vi "variantCtrlIoAddress.vi"(4 "isRequired (T)":bool=TRUE, 6 "menu in (get)":enum16{"get", "set"}(ring), 8 "error in":errorcluster, 9 "ADDR":T1 format="%04d", 11 "variant in":variant) -> (0 "error out":errorcluster, 1 "ADDR":T1 format="%04d", 2 "isFound?":bool, 3 "variant out":variant)   [LabVIEW 2024]
uses:
  controls/type.address.ctl
  controls/typeEngErrorCodes.ctl
panel:
  out "spreadsheet string":string
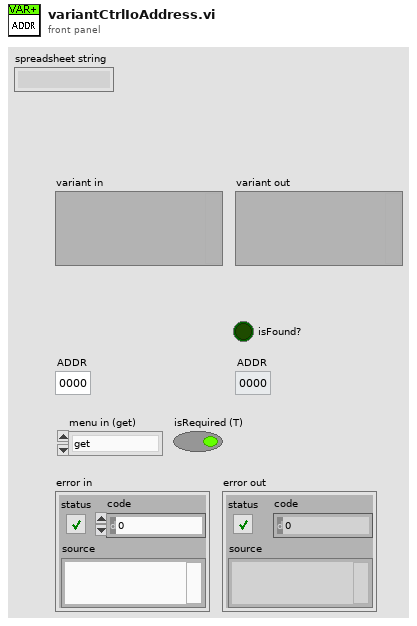
[diagram p1: front panel]
types:
  T1 = typedef "type.address.ctl" = u16
  T2 = typedef "typeEngErrorCodes.ctl" = u16
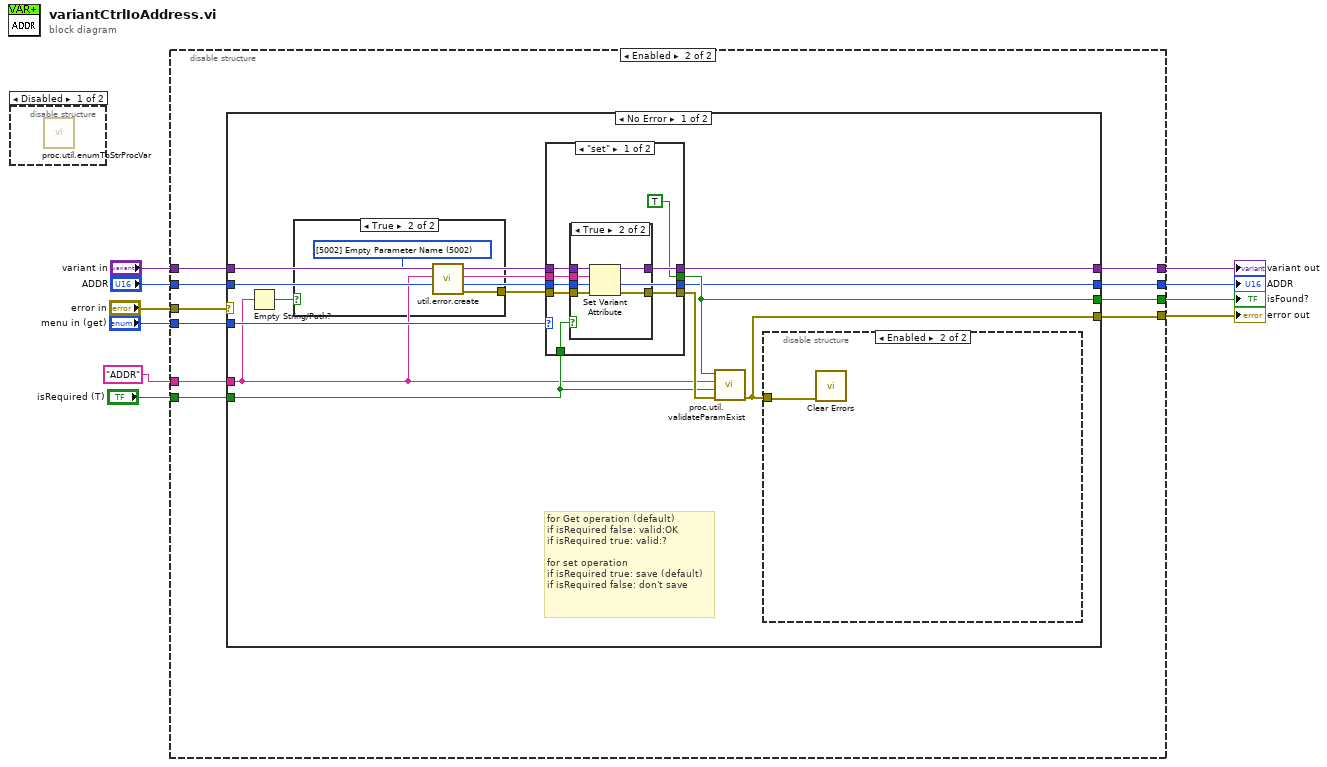
[diagram p0: block diagram]
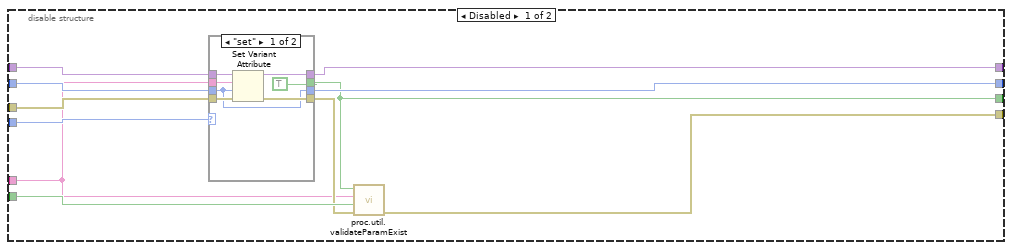
[diagram p2: hidden frame]
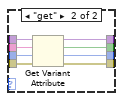
[diagram p3: hidden frame]
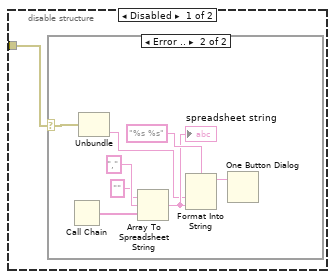
[diagram p5: hidden frame]
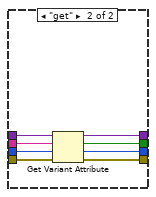
[diagram p8: hidden frame]
diagram:
  n1 = disable-structure shown="Disabled" {
    frame Disabled {
      n2 = call "proc.util.enumToStrProcVar.vi"() -> ()  [unwired: 11 in, 1 out]
    }
    frame Enabled {
    }
  }
  n3 = disable-structure shown="Enabled" {
    disable-tunnel: "error in" -> [w21 w43]
    disable-tunnel: "ADDR" -> [w20 w42]
    disable-tunnel: "variant in" -> [w19 w41]
    disable-tunnel: [w18 w40] -> w7
    disable-tunnel: "menu in (get)" -> [w17 w44]
    disable-tunnel: [w16 w38] -> w5
    disable-tunnel: "isRequired (T)" -> [w15 w45]
    disable-tunnel: [w14 w39] -> w3
    disable-tunnel: [w12 w37] -> w2
    disable-tunnel: "ADDR" ("name in") -> [w11 w46]
    frame Disabled {
      n4 = case shown="\"set\"" w17 {
        tunnel: w21 -> [w28 w36]
        tunnel: w20 -> [w23 w35]
        tunnel: w19 -> [w27 w34]
        tunnel: [w26 w33] -> w13
        tunnel: [TRUE w32] -> w14
        tunnel: [w25 w31] -> w18
        tunnel: w11 -> [w24 w30]
        tunnel: [w23 w29] -> w16
        frame "set" {
          n5 = Set Variant Attribute(Variant=w27, name=w24, value=w23, error in=w28) -> (Variant out=w25:variant, error out=w26:errorcluster)  [unwired: 1 out]
        }
        frame "get" {
          n6 = Get Variant Attribute(Variant=w34, name=w30, default value (empty Variant)=w35, error in=w36) -> (duplicate Variant=w31:variant, found=w32:bool, value=w29:T1, error out=w33:errorcluster)
        }
      }
      n7 = call "proc.util.validateParamExist.vi"("error in"=w13, "isRequired"=w15, "Param Label"=w11, "isFound"=w14) -> ("error out"=w12:errorcluster)  [unwired: 7 in]
    }
    frame Enabled {
      n8 = case shown="No Error" w43 {
        selector: w43 -> [_ w97]
        tunnel: w42 -> [w58 w95]
        tunnel: w41 -> [w57 w96]
        tunnel: [w51 w96] -> w40
        tunnel: w44 -> [w56 _]
        tunnel: [w50 w95] -> w38
        tunnel: w45 -> [w52 _]
        tunnel: [w55 _] -> w39
        tunnel: w46 -> [w49 _]
        tunnel: [w53 w97] -> w37
        frame No Error {
          # "for Get operation (default)\nif isRequired false: valid:OK\nif isRequired true: valid:?\n\nfor set operation\nif isRequired true: save (default)\nif isRequired false: don't save"
          n9 = Empty String/Path?(string/path=w49) -> (empty?=w48:bool)
          n10 = case shown="True" w48 {
            tunnel: [_ w59] -> w47
            frame False {
            }
            frame True {
              w60 = T2 5002 items=["[5000] Missing Function Arguments"=5000, "[5001] Incorrect Function Arguments"=5001, "[5002] Empty Parameter Name"=5002, "[5010] Not Found"=5010] ("Ring")
              n11 = call "util.error.create.vi"("Ring"=w60) -> ("error out"=w59:errorcluster)  [unwired: 9 in, 1 out]
            }
          }
          n12 = case shown="\"set\"" w56 {
            tunnel: w47 -> [w78 w94]
            tunnel: w58 -> [w73 w93]
            tunnel: w57 -> [w77 w92]
            tunnel: [w76 w91] -> w54
            tunnel: [TRUE w90] -> w55
            tunnel: [w75 w89] -> w51
            tunnel: w49 -> [w74 w88]
            tunnel: [w73 w87] -> w50
            tunnel: w52 -> [w71 _]
            frame "set" {
              n13 = case shown="True" w71 {
                tunnel: w78 -> [w79 w86]
                tunnel: w77 -> [w80 w85]
                tunnel: [w79 w84] -> w76
                tunnel: [w80 w83] -> w75
                tunnel: w74 -> [_ w82]
                tunnel: w73 -> [_ w81]
                frame False {
                }
                frame True {
                  n14 = Set Variant Attribute(Variant=w85, name=w82, value=w81, error in=w86) -> (Variant out=w83:variant, error out=w84:errorcluster)  [unwired: 1 out]
                }
              }
            }
            frame "get" {
              n15 = Get Variant Attribute(Variant=w92, name=w88, default value (empty Variant)=w93, error in=w94) -> (duplicate Variant=w89:variant, found=w90:bool, value=w87:T1, error out=w91:errorcluster)
            }
          }
          n16 = call "proc.util.validateParamExist.vi"("error in"=w54, "isRequired"=w52, "Param Label"=w49, "isFound"=w55) -> ("error out"=w53:errorcluster)  [unwired: 7 in]
          n17 = disable-structure shown="Enabled" {
            disable-tunnel: w53 -> [w61 w70]
            frame Disabled {
              n18 = case shown="Error .." w61 {
                selector: w61 -> [_ w69]
                frame No Error {
                }
                frame Error {
                  n19 = Call Chain() -> (call chain=w68:string[])
                  n20 = Unbundle(w69) -> ("source"=w62:string)  [unwired: 2 out]
                  n21 = Array To Spreadsheet String(delimiter (Tab)=",", array=w68, 3:"" ("format string")) -> (spreadsheet string=w64:string)
                  "spreadsheet string" <- w64
                  n22 = Format Into String(format string="%s %s", w62, w64) -> (resulting string=w63:string)  [unwired: 2 in, 1 out]
                  n23 = One Button Dialog(message=w63) -> ()  [unwired: 1 in, 1 out]
                }
              }
            }
            frame Enabled {
              n24 = call <vilib>:"Clear Errors.vi"("error in (no error)"=w70) -> ()  [unwired: 5 in, 2 out]
            }
          }
        }
        frame Error {
        }
      }
    }
  }
  "error out" <- w2
  "isFound?" <- w3
  "variant out" <- w7
  "ADDR" <- w5
